vi "Gyro Loop.vi"() -> (0 "Active Gyro":string)   [LabVIEW 2015, in "Apple Pi Gyro Library.lvlib"]
uses:
  Apple Pi Gyro Library.lvlib
  <vilib>/Rock Robotics/Network Tables/NT Read Number.vi
  ADI MXP IMU/ADI MXP IMU/FRC_ADIS16448_IMU.lvlib
  SimpleGyro ADXRS453/SimpleGyro.lvlib
panel:
  # "Place me in Periodic Tasks\n\nAll Done :D"
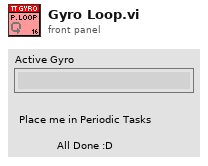
[diagram p1: front panel]
types:
  T1 = typedef "Apple Pi Gyro Library.lvlib/SimpleGyro.lvlib/WPI_SimpleGyroDevRef.ctl" = cluster{"DevStatus":errorcluster, "Handle":i32, "SPI Bus":T2, "Device Found":bool, "Sample Rate":dbl}
  T2 = typedef "spi_bus.ctl" = enum16{"SPI On-Board, CS0", "SPI On-Board, CS1", "SPI On-Board, CS2", "SPI On-Board, CS3", "SPI MXP", "Invalid"}
  T3 = typedef "Apple Pi Gyro Library.lvlib/FRC_ADIS16448_IMU.lvlib/WPI_IMU_ADIS16448_InterruptDevRef.ctl" = cluster{"ADI IMU DevRef":T4, "InterruptRef":T5}
  T4 = typedef "Apple Pi Gyro Library.lvlib/FRC_ADIS16448_IMU.lvlib/WPI_IMU_ADIS16448_IMUDevRef.ctl" = cluster{"DevStatus":errorcluster, "Handle":i32, "SPI Bus":T2, "Device Found":bool, "Device Ready":bool, "Yaw Axis":enum16{"X", "Y", "Z"}, "AHRS Algorithm":enum16{"Complementary", "Madgwick"}, "Serial":u16, "Lot ID 2":u16, "Lot ID 1":u16, "Product ID":u16}
  T5 = typedef "WPI_InterruptRef.ctl" = cluster{"DevStatus":errorcluster, "InterruptIndex":T6}
  T6 = typedef "FPGA_InterruptIndex.ctl" = enum8{"0", "1", "2", "3", "4", "5", "6", "7", "Invalid"}
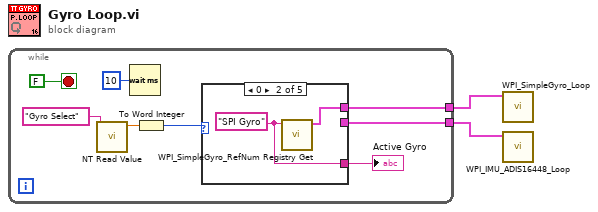
[diagram p0: block diagram]
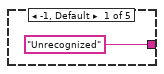
[diagram p2: hidden frame]
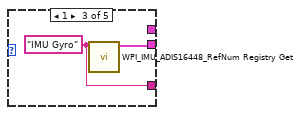
[diagram p3: hidden frame]
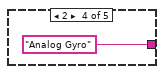
[diagram p4: hidden frame]
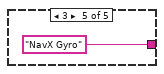
[diagram p5: hidden frame]
diagram:
  n1 = while {
    tunnel: [w5] -> w2
    tunnel: [w4] -> w1
    stop <- FALSE stop-if-true
    n2 = call-poly <vilib>:"NT Read Value.vi"("Name"="Gyro Select") -> ("Numeric"=w6:dbl)  [unwired: 9 in, 1 out]
    n3 = Wait (ms)(milliseconds to wait=u32 10) -> ()  [unwired: 1 out]
    n4 = To Word Integer(number=w6) -> (16bit integer=w3:i16)
    n5 = case shown="0" w3 {
      tunnel: ["Unrecognized" ("refnum name") w13 w15 "Analog Gyro" "NavX Gyro"] -> w9
      tunnel: [_ _ w14 _ _] -> w5
      tunnel: [_ w12 _ _ _] -> w4
      frame -1, Default {
      }
      frame 0 {
        w13 = "SPI Gyro" ("refnum name")
        n6 = call "WPI_SimpleGyro_RefNum Registry Get.vi"("refnum name"=w13) -> ("SimpleGyroDevRef"=w12:T1)  [unwired: 9 in, 1 out]
      }
      frame 1 {
        w15 = "IMU Gyro" ("refnum name")
        n7 = call "WPI_IMU_ADIS16448_RefNum Registry Get.vi"("refnum name"=w15) -> ("ADI IMU Interrupt DevRef"=w14:T3)  [unwired: 9 in, 1 out]
      }
      frame 2 {
      }
      frame 3 {
      }
    }
    "Active Gyro" <- w9
  }
  n8 = call "WPI_SimpleGyro_Loop.vi"("SimpleGyroDevRef"=w1) -> ()  [unwired: 10 in, 1 out]
  n9 = call "WPI_IMU_ADIS16448_Loop.vi"("ADI IMU Interrupt DevRef"=w2) -> ()  [unwired: 9 in, 2 out]
